vi "DHE_DRV_clear_progress_buf.vi"(0 "fd":i32, 11 "error in (no error)":errorcluster) -> (4 "fd":i32, 8 "return value":i32, 15 "error out":errorcluster)   [LabVIEW 2016]
doc: "This VI closes the I/O interface with the instrument."
uses:
  c/lib/libarcDHE.so
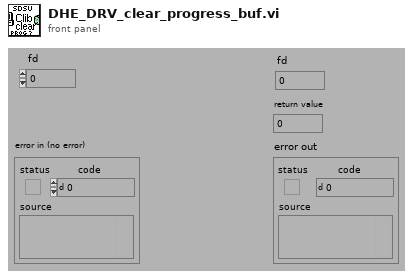
[diagram p1: front panel]
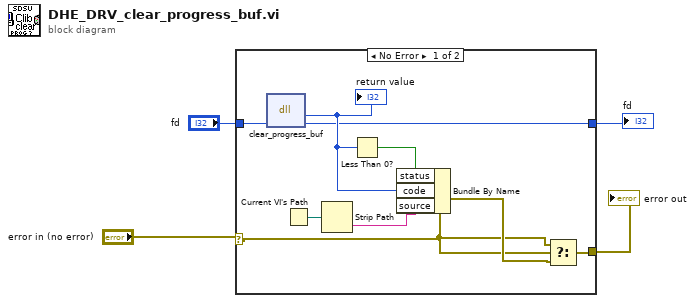
[diagram p0: block diagram]
diagram:
  n1 = case shown="No Error" "error in (no error)" {
    selector: "error in (no error)" -> [w6 w15]
    tunnel: "fd" -> [w13 w14]
    tunnel: [w7 w15] -> w3
    tunnel: [w5 w14] -> w1
    frame No Error {
      n2 = dll-call lib="home/simager/panview/PAN/Modules/SDSU/private/c/lib/libarcDHE.so" fn="clear_progress_buf"("fd"=w13) -> (w11:i32, "fd"=w5:i32)  [unwired: 3 in, 2 out]
      "return value" <- w11
      n3 = Current VI's Path() -> (path=w10:path)
      n4 = Strip Path(path=w10) -> (name=w9:string)  [unwired: 1 out]
      n5 = Less Than 0?(x=w11) -> (x < 0?=w12:bool)
      n6 = Bundle By Name(cluster=w6, "status"=w12, "code"=w11, "source"=w9) -> (w8:errorcluster)
      n7 = Select(t=w6, s=w6, f=w8) -> (s? t:f=w7:errorcluster)
    }
    frame Error {
    }
  }
  "error out" <- w3
  "fd" <- w1
